vi "dfd_Convert MRate Filter to String.vi"(5 "indent order":i32, 7 "format string":string="%-+022.16e", 11 "multirate filter in":T1={"mMRate_Structure"=enum."FIR", "mMRate_Mode"=0, "mMRate_Factor"=1, "mMRate_FIRParams"={"mMRate_FIR_H"=[], "mMRate_FIR_IsNyquist?"=FALSE, "mMRate_FIR_IsSymmetric?"=FALSE}, "mMRate_CICParams"={"mMRate_CIC_#Stage"=2, "mMRate_CIC_Lag"=1, "mMRate_CIC_Type"=enum."Lowpass"}, "mMRate_Order"=0, "mMRate_Version"="2.0", "mMRate_Comments"="", "mMRate_RationalFactor"={"mMRate_L"=-1, "mMRate_M"=-1}, "mMRate_Fs"=1.0, "mMRate_Quantized?"=FALSE, "mMRate_QFilterGain"=1.0, "mMRate_CoefWl"=16, "mMRate_Scaling"={"mMRate_ScaleByPowerOf2?"=FALSE, "mMRate_ScaleType"=enum."Time Domain 1-Norm"}, "mMRate_InputWl"=16, "mMRate_OutputWl"=16, "mMRate_OutputMode"=enum."Nearest", "mMRate_MultMode"=enum."Truncated", "mMRate_BitPruning"=FALSE, "mMRate_GainWl"=16, "mMRate_OutputFwl"=0, "mMRate_SumIwl"=0, "mMRate_InputIwl "=16, "mMRate_SumWl"=32, "mMRate_CoefIwl"=0} {"mMRate_SumWl" min=1 max=32 step=1; "mMRate_InputIwl" min=1 max=32 step=1; "mMRate_GainWl" min=1 max=32 step=1; "mMRate_OutputWl" min=1 max=32 step=1; "mMRate_InputWl" min=1 max=32 step=1; "mMRate_CoefWl" min=1 max=32 step=1; "mMRate_Mode" items=["Default"=-1, "No Rate Change"=0, "Interpolation"=1, "Decimation"=2, "Interpolated"=3, "Rational"=4]}) -> (3 "xml string":string)   [LabVIEW 2017, in "NI_DigFilter_Process.lvlib"]
uses:
  <vilib>/addons/Digital Filter Design/NI_DigFilter_Process.lvlib
  <vilib>/addons/Digital Filter Design/_Objects.llb/DFD Multirate Filter Obj.ctl
  <vilib>/addons/Digital Filter Design/_Objects.llb/DFD Multirate Mode.ctl
  <vilib>/addons/Digital Filter Design/_Objects.llb/DFD Coef Norm Type.ctl
  <vilib>/addons/Digital Filter Design/_Objects.llb/DFD Round-off Mode.ctl
  <vilib>/addons/Digital Filter Design/_Objects.llb/DFD FXP MRate Multiply Mode.ctl
  <vilib>/addons/Digital Filter Design/NI_DigFilterLicensed.lvlib
panel:
  in  "width (-)":i16=8
  out "error out":errorcluster
  in  "error in (no error)":errorcluster
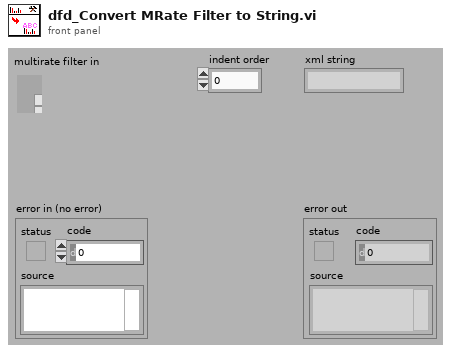
[diagram p1: front panel]
types:
  T1 = typedef "NI_DigFilterLicensed.lvlib/DFD Multirate Filter Obj.ctl" = cluster{"mMRate_Structure":enum16{"CIC", "FIR", "IIR", "Lattice"}, "mMRate_Mode":T2, "mMRate_Factor":i32, "mMRate_FIRParams":cluster{"mMRate_FIR_H":dbl[], "mMRate_FIR_IsNyquist?":bool, "mMRate_FIR_IsSymmetric?":bool}, "mMRate_CICParams":cluster{"mMRate_CIC_#Stage":i32, "mMRate_CIC_Lag":i32, "mMRate_CIC_Type":enum16{"Lowpass", "Highpass"}}, "mMRate_Order":i32, "mMRate_Version":string, "mMRate_Comments":string, "mMRate_RationalFactor":cluster{"mMRate_L":i32, "mMRate_M":i32}, "mMRate_Fs":dbl, "mMRate_Quantized?":bool, "mMRate_QFilterGain":dbl, "mMRate_CoefWl":i16, "mMRate_Scaling":cluster{"mMRate_ScaleByPowerOf2?":bool, "mMRate_ScaleType":T3}, "mMRate_InputWl":i16, "mMRate_OutputWl":i16, "mMRate_OutputMode":T4, "mMRate_MultMode":T5, "mMRate_BitPruning":bool, "mMRate_GainWl":i16, "mMRate_OutputFwl":i16, "mMRate_SumIwl":i16, "mMRate_InputIwl ":i16, "mMRate_SumWl":i16, "mMRate_CoefIwl":i16}
  T2 = typedef "NI_DigFilterLicensed.lvlib/DFD Multirate Mode.ctl" = i16
  T3 = typedef "NI_DigFilterLicensed.lvlib/DFD Coef Norm Type.ctl" = enum16{"No Norm", "Time Domain 1-Norm", "Time Domain 2-Norm", "Time Domain Inf-Norm"}
  T4 = typedef "NI_DigFilterLicensed.lvlib/DFD Round-off Mode.ctl" = enum16{"Nearest", "Truncation"}
  T5 = typedef "NI_DigFilterLicensed.lvlib/DFD FXP MRate Multiply Mode.ctl" = enum16{"Truncated", "Full"}
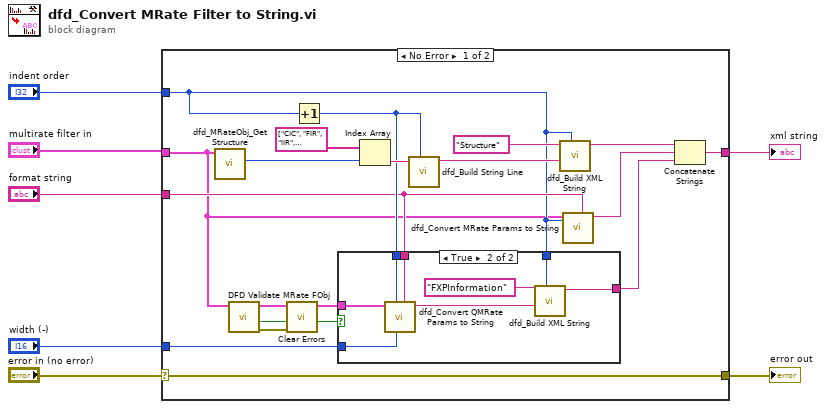
[diagram p0: block diagram]
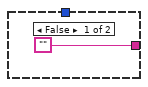
[diagram p2: hidden frame]
diagram:
  n1 = case shown="No Error" "error in (no error)" {
    selector: "error in (no error)" -> [w22 w35]
    tunnel: "multirate filter in" -> [w12 _]
    tunnel: "format string" -> [w16 _]
    tunnel: [w23 _] -> w6
    tunnel: [w22 w35] -> w5
    tunnel: "indent order" -> [w14 _]
    tunnel: "width (-)" -> [w18 _]
    frame No Error {
      n2 = call <vilib>:"dfd_MRateObj_Get Structure.vi"("multirate filter in"=w12) -> ("structure"=w13:enum16{"CIC", "FIR", "IIR", "Lattice"})  [unwired: 10 out]
      n3 = call <vilib>:"DFD Validate MRate FObj.vi"("multirate filter in"=w12) -> ("error out"=w9:errorcluster, "is valid FXP?"=w10:bool, "multirate filter out"=w11:T1)  [unwired: 1 in, 7 out]
      n4 = call <vilib>:"Clear Errors.vi"("error in (no error)"=w9) -> ()  [unwired: 1 in, 6 out]
      n5 = Increment(x=w14) -> (x+1=w17:i32)
      n6 = case shown="True" w10 {
        tunnel: ["" w32] -> w19
        tunnel: w18 -> [_ w31]
        tunnel: w11 -> [_ w30]
        tunnel: w17 -> [_ w29]
        tunnel: w16 -> [_ w28]
        tunnel: w14 -> [_ w27]
        frame False {
        }
        frame True {
          n7 = call <vilib>:"dfd_Convert QMRate Params to String.vi"("format string"=w28, "width (-)"=w31, "indent order"=w29, "multirate filter in"=w30) -> ("string"=w33:string)  [unwired: 7 out]
          n8 = call <vilib>:"dfd_Build XML String.vi"("indent order"=w27, "string in"=w33, "element name"="FXPInformation") -> ("xml string out"=w32:string)  [unwired: 1 in, 7 out]
        }
      }
      n9 = Index Array(array=string[] ["CIC", "FIR", "IIR", "Lattice"] ("structure"), index=w13) -> (element=w20:string)
      n10 = call <vilib>:"dfd_Build String Line.vi"("indent order"=w17, "string"=w20) -> ("string line"=w21:string)  [unwired: 9 out]
      n11 = call <vilib>:"dfd_Build XML String.vi"("indent order"=w14, "string in"=w21, "element name"="Structure") -> ("xml string out"=w24:string)  [unwired: 1 in, 7 out]
      n12 = call <vilib>:"dfd_Convert MRate Params to String.vi"("format string"=w16, "indent order"=w14, "multirate filter in"=w12) -> ("string"=w15:string)  [unwired: 1 in, 7 out]
      n13 = Concatenate Strings(w24, w15, w19) -> (w23:string)
    }
    frame Error {
    }
  }
  "xml string" <- w6
  "error out" <- w5
